vi "udp-connectie - kopie.vi"() -> ()   [LabVIEW 2019]
panel:
  in  "stop":bool
  out "port":u16
  in  "data in":string
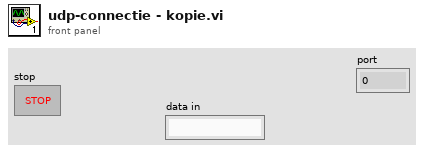
[diagram p1: front panel]
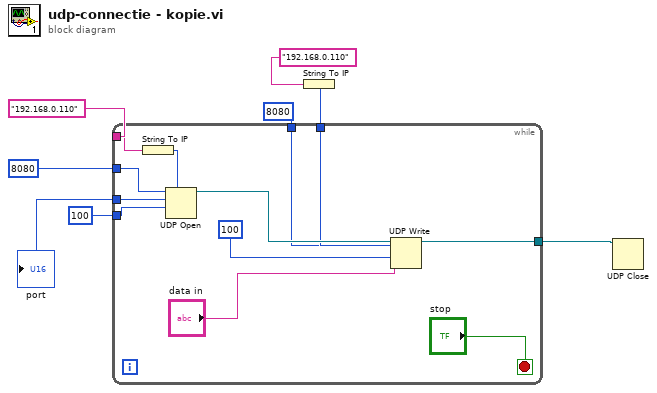
[diagram p0: block diagram]
diagram:
  n1 = String To IP(1:"192.168.0.110") -> (0:w5:u32)
  n2 = while {
    tunnel: 8080 -> [w19]
    tunnel: "192.168.0.110" -> [w18]
    tunnel: w5 -> [w16]
    tunnel: 8080 -> [w15]
    tunnel: 100 ("timeout ms (25000)") -> [w14]
    tunnel: [w11] -> w2
    tunnel: [w10] -> w1
    stop <- "stop" stop-if-true
    n3 = String To IP(1:w18) -> (0:w20:u32)
    n4 = UDP Open(7:w20, 9:w14, 11:w19) -> (port=w17:refnum<k16>, 2:w11:u16)  [unwired: 2 in, 1 out]
    n5 = UDP Write(address=w16, port or service name=w15, connection ID=w17, data in="data in", 9:100 ("timeout ms (25000)")) -> (3:w10:refnum<k16>)  [unwired: 1 in, 1 out]
  }
  "port" <- w2
  n6 = UDP Close(connection ID=w1) -> ()  [unwired: 1 in, 2 out]
